vi "GetDataTrProcModeStr.vi"(8 "错误输入（无错误）":errorcluster, 9 "数据传输模式":u8, 10 "字符串空间大小":u32, 11 "字符串地址":string) -> (0 "错误输出":errorcluster, 3 "字符串地址":string)   [LabVIEW 2014]
uses:
  X86Dll/ZXUTConfigMgr.dll
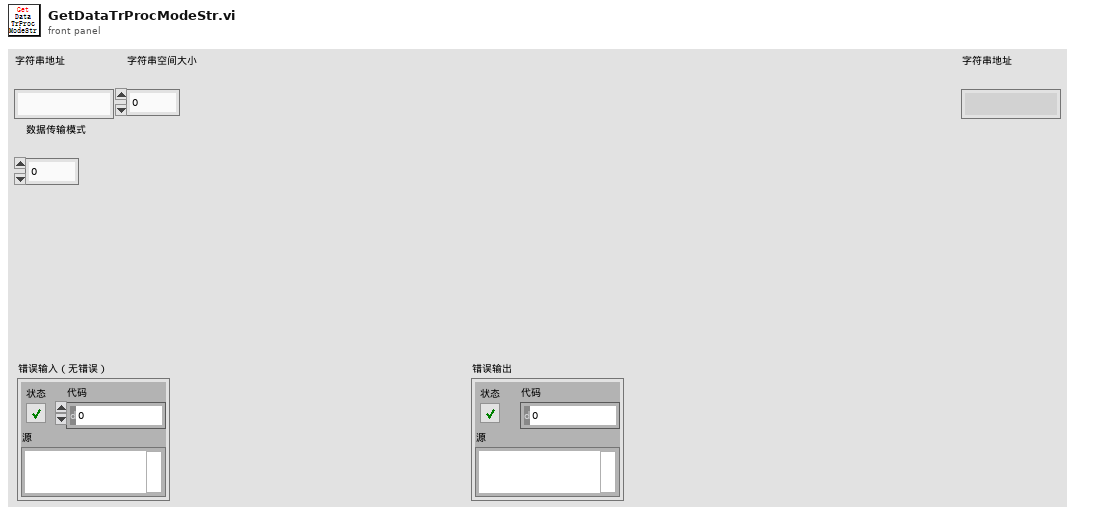
[diagram p1: front panel]
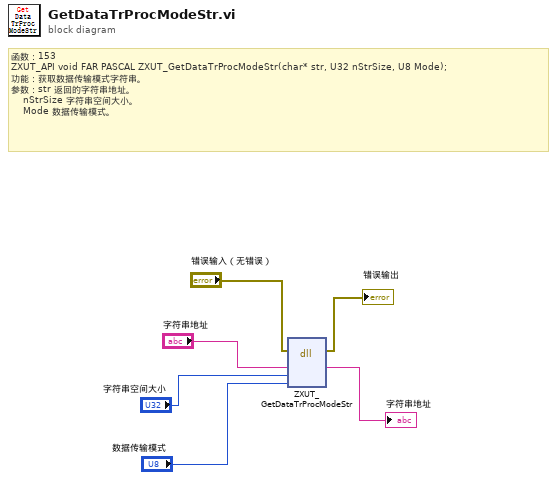
[diagram p0: block diagram]
diagram:
  # "函数：153\nZXUT_API void\tFAR PASCAL ZXUT_GetDataTrProcModeStr(char* str, U32 nStrSize, U8 Mode);\n功能：获取数据传输模式字符串。\n参数：str 返回的字符串地址。\n\t   nStrSize 字符串空间大小。\n\t   Mode 数据传输模式。"
  n1 = dll-call lib="D:/Software/Utrasonic on-line monitoring/X86Dll/ZXUTConfigMgr.dll" fn="ZXUT_GetDataTrProcModeStr"(error in="错误输入（无错误）", "str"="字符串地址", "nStrSize"="字符串空间大小", "Mode"="数据传输模式") -> (error out=→"错误输出":errorcluster, "str"=→"字符串地址":string)  [unwired: 5 in, 1 out]
